vi "Main.vi"() -> ()   [LabVIEW 2019]
uses:
  MoveoSerialClass/MoveoSerial.lvclass
panel:
  in  "SendString":string="M110"
  out "Verknüpfter String":string
  in  "Boolesch":bool
  out "error out":errorcluster caption="Fehler (Ausgang)"
  in  "VISA resource name":refnum<visa-resource-name>
  in  "Stopp":bool
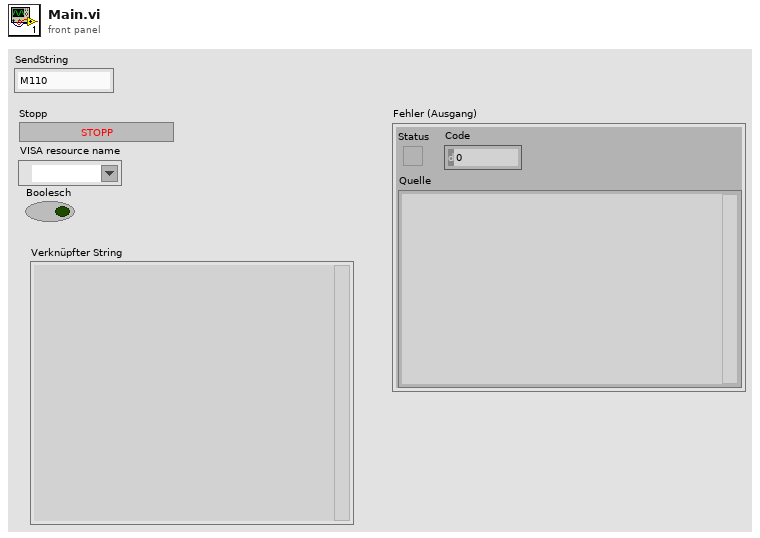
[diagram p1: front panel]
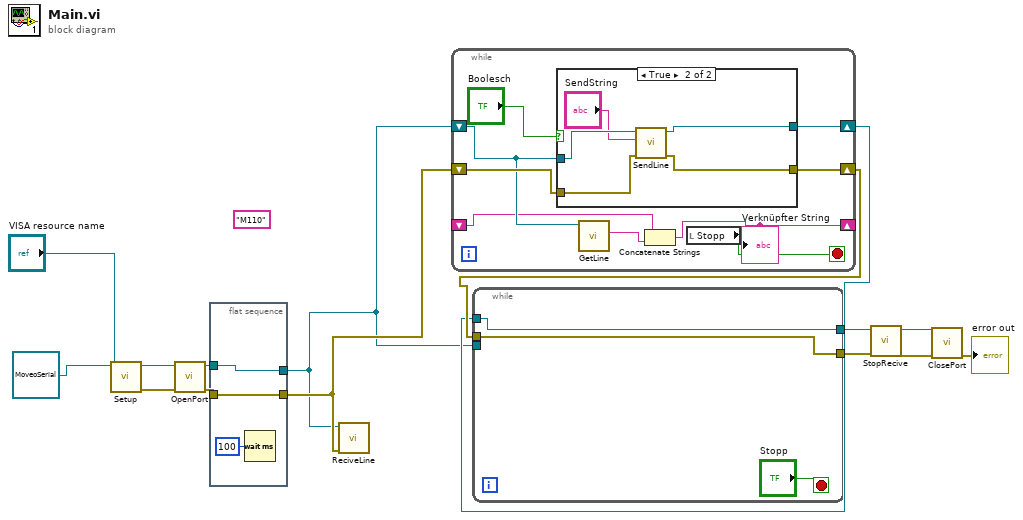
[diagram p0: block diagram]
diagram:
  (unwired) "M110" ("SendString")
  n1 = call-dynamic "Setup.vi"("VISA resource name"="VISA resource name", "MoveoSerial Eingang"=refnum<class "MoveoSerial.lvclass"> refnum ("MoveoSerial.lvclass")) -> ("error out"=w9:errorcluster, "MoveoSerial Ausgang"=w14:refnum<class "MoveoSerial.lvclass">)  [unwired: 8 in]
  n2 = call-dynamic "OpenPort.vi"("error in (no error)"=w9, "MoveoSerial Eingang"=w14) -> ("error out"=w3:errorcluster, "MoveoSerial Ausgang"=w4:refnum<class "MoveoSerial.lvclass">)  [unwired: 8 in]
  n3 = flat-sequence {
    tunnel: [w18] -> w1
    tunnel: w4 -> [w18]
    tunnel: [w17] -> w2
    tunnel: w3 -> [w17]
    frame #0 {
      n4 = Wait (ms)(milliseconds to wait=u32 100 ("Zu wartende ms")) -> ()  [unwired: 1 out]
    }
  }
  n5 = call-dynamic "ReciveLine.vi"("error in (no error)"=w2, "MoveoSerial Eingang"=w1) -> ()  [unwired: 8 in, 2 out]
  n6 = while {
    shift-right: [w24] -> w5
    shift-left: w1 -> [w22]
    shift-right: [w23] -> w6
    shift-left: w2 -> [w25]
    shift-right: [w20] -> _
    shift-left: _ -> [w19]
    stop <- w27 stop-if-true
    n7 = case shown="True" "Boolesch" {
      tunnel: w22 -> [w29 w34]
      tunnel: w25 -> [w28 w33]
      tunnel: [w29 w32] -> w24
      tunnel: [w28 w31] -> w23
      frame False {
      }
      frame True {
        n8 = call-dynamic "SendLine.vi"("error in (no error)"=w33, "SendString"="SendString", "MoveoSerial Eingang"=w34) -> ("error out"=w31:errorcluster, "MoveoSerial Ausgang"=w32:refnum<class "MoveoSerial.lvclass">)  [unwired: 7 in]
      }
    }
    n9 = call-dynamic "GetLine.vi"("MoveoSerial Eingang"=w22) -> ("RecivedLine"=w21:string)  [unwired: 8 in, 2 out]
    n10 = Concatenate Strings(w19, w21) -> (w20:string)
    "Verknüpfter String" <- w20
    n11 = local read "Stopp"() -> (w27:bool)
  }
  n12 = while {
    tunnel: w5 -> [w36]
    tunnel: [w36] -> w13
    tunnel: [w35] -> w10
    tunnel: w6 -> [w35]
    tunnel: w1 -> [_]
    stop <- "Stopp" stop-if-true
  }
  n13 = call-dynamic "StopRecive.vi"("error in (no error)"=w10, "MoveoSerial Eingang"=w13) -> ("error out"=w11:errorcluster, "MoveoSerial Ausgang"=w12:refnum<class "MoveoSerial.lvclass">)  [unwired: 8 in]
  n14 = call-dynamic "ClosePort.vi"("error in (no error)"=w11, "MoveoSerial Eingang"=w12) -> ("error out"=→"error out":errorcluster)  [unwired: 8 in, 1 out]
